vi "Poll.Main.vi"(8 "error in (no error)":errorcluster, 10 "Paramaters":variant, 11 "Process":refnum<class "Process.lvclass">) -> ()   [LabVIEW 2015, in "OPC UA Client Engine.lvlib"]
uses:
  OPC UA Client Engine.lvlib
  <vilib>/NI/NIVS Inline Async API/_VS Inline Async API/Process/Process.lvclass
  Types/Poll.Parameters.ctl
  Shared/Compiled.Settings.ctl
  Shared/OPCConnection.Properties.ctl
  Shared/Poll.ListProperties.ctl
  Shared/Tag.WriteProperties.Info.ctl
  Shared/Tags.ReadWriteRefs.ctl
  <vilib>/NI Veristand/Custom Device API/Data Reference.ctl
  <vilib>/NI Veristand/Custom Device API/Custom Device Target Type.ctl
  <vilib>/NI/NIVS Inline Async API/_Data Access Engine/Access Type Classes/Write/Write.lvclass/Write.ctl
  <vilib>/NI/NIVS Inline Async API/_VS Inline Async API/Process/Process.lvclass/Process.ctl
  Shared/DataRefs.Location.ctl
  <vilib>/NI/NIVS Inline Async API/_Data Access Engine/Data Access Engine/Methods/Write.Data.vi
  <vilib>/NI/NIVS Inline Async API/_VS Inline Async API/Error Handling Process/SubVIs/Error.ConvertArray.vi
  <vilib>/NI/NIVS Inline Async API/_Data Access Engine/Access Type Classes/Write/Write.ProcessData.vi
  <vilib>/OPCUA/client/Write DateTime Array.vi
  <vilib>/OPCUA/client/Write Double Array.vi
  <vilib>/OPCUA/client/Write Float Array.vi
  <vilib>/OPCUA/client/Write UInt64 Array.vi
  <vilib>/OPCUA/client/Write Int64 Array.vi
  <vilib>/OPCUA/client/Write UInt32 Array.vi
  <vilib>/OPCUA/client/Write Int32 Array.vi
  <vilib>/OPCUA/client/Write UInt16 Array.vi
  <vilib>/OPCUA/client/Write Int16 Array.vi
  <vilib>/OPCUA/client/Write Byte Array.vi
  <vilib>/OPCUA/client/Write SByte Array.vi
  <vilib>/OPCUA/client/Write Bool Array.vi
  <vilib>/OPCUA/client/Write DateTime.vi
  <vilib>/OPCUA/client/Write Double.vi
  <vilib>/OPCUA/client/Write Float.vi
  <vilib>/OPCUA/client/Write UInt64.vi
  <vilib>/OPCUA/client/Write Int64.vi
  <vilib>/OPCUA/client/Write UInt32.vi
  <vilib>/OPCUA/client/Write Int32.vi
  <vilib>/OPCUA/client/Write UInt16.vi
  <vilib>/OPCUA/client/Write Int16.vi
  <vilib>/OPCUA/client/Write Byte.vi
  <vilib>/OPCUA/client/Write SByte.vi
  <vilib>/OPCUA/client/Write Bool.vi
  <vilib>/OPCUA/NI OPC UA Client.lvlib
  Shared/OPC UA Client Shared.lvlib
  <vilib>/NI Veristand/Custom Device Tools/Custom Device Utility Library/Custom Device Utility Library.lvlib
  <vilib>/NI VeriStand/Custom Device API/Custom Device API.lvlib
  <vilib>/NI/NIVS Inline Async API/_Data Access Engine/Data Access Engine/Data Access Engine.lvclass
panel:
  out "Read Code":i32
  out "Write Code":i32
  out "Read Table":variant
  out "Write Table":variant
  out "error out":errorcluster
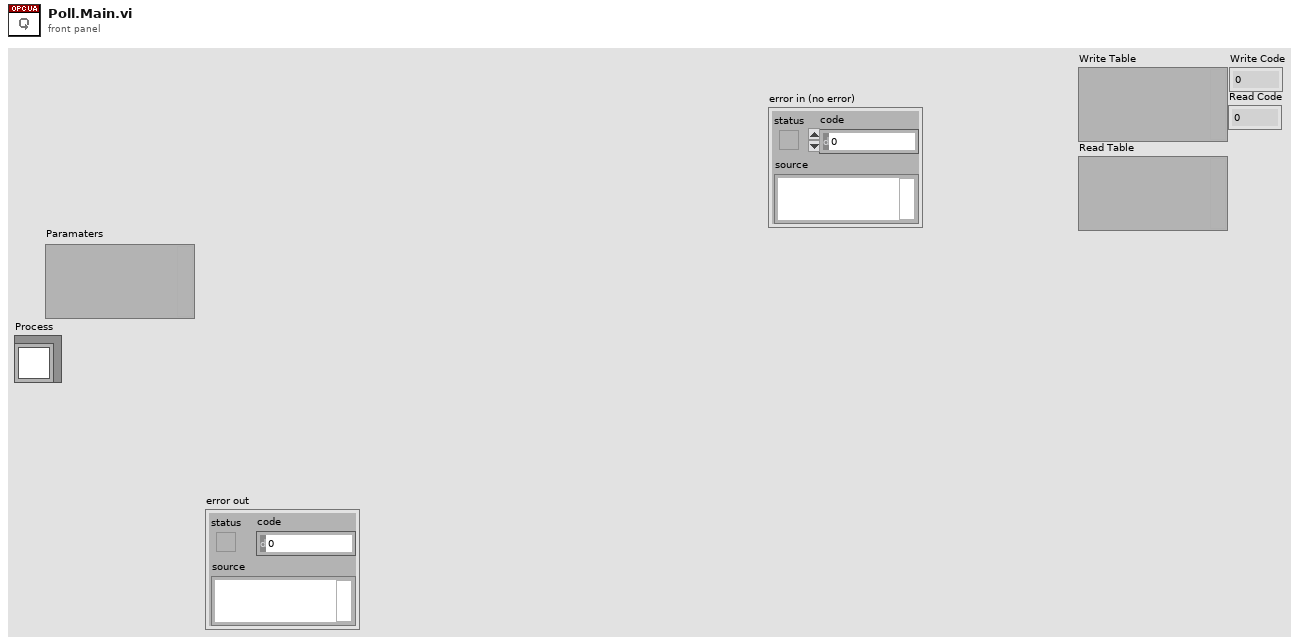
[diagram p1: front panel]
types:
  T1 = typedef "OPC UA Client Engine.lvlib/Poll.Parameters.ctl" = cluster{"Settings":T2, "WriteData":refnum<k33>, "ReadData":refnum<k33>, "WriteUpdate":refnum<k33>, "ReadUpdate":refnum<k33>, "Target Type":T8}
  T2 = typedef "OPC UA Client Shared.lvlib/Compiled.Settings.ctl" = cluster{"Connection.Properties":T3, "PollEngine.Settings":T4[], "LUT":variant, "Write Locations":T5[], "TotalTags":u32, "Data Refs":T6}
  T3 = typedef "OPC UA Client Shared.lvlib/OPCConnection.Properties.ctl" = cluster{"Server IP Address":string, "Server Port":u16, "Message Mode":enum16{"None", "Sign", "Sign and Encrypt"}, "Security":enum16{"Basic256", "Basic128Rsa15"}, "User Name":string, "Password":string, "Client Certificate":path, "Server Certificate":path, "Server Certificate (RT)":path, "Client Certificate (RT)":path}
  T4 = typedef "OPC UA Client Shared.lvlib/Poll.ListProperties.ctl" = cluster{"Poll Rate":dbl, "Tags":string[]}
  T5 = typedef "OPC UA Client Shared.lvlib/Tag.WriteProperties.Info.ctl" = cluster{"Path":string, "Offset":i32, "Length":i32, "DataType":u32}
  T6 = typedef "OPC UA Client Shared.lvlib/Tags.ReadWriteRefs.ctl" = cluster{"Read Refs":T7[], "Read Values":dbl[], "Read?":bool[], "Access":enum8{"Null", "Read", "Write", "Read&Write"}[], "Write Refs":T7[], "Write Values":dbl[], "Write?":bool[], "Write Only Location":u32, "Write? Reset":bool[]}
  T7 = typedef "Custom Device API.lvlib/Data Reference.ctl" = i32
  T8 = typedef "Custom Device API.lvlib/Custom Device Target Type.ctl" = enum16{"PharLap", "VxWorks", "Windows", "Linux_32_ARM", "Linux_x64"}
  T9 = typedef "OPC UA Client Shared.lvlib/DataRefs.Location.ctl" = cluster{"Offset":i32, "Length":i32}
  T10 = typedef "OPC UA Client Engine.lvlib/Poll.StateVariables.ctl" = cluster{"SubscriptionIDs":u32[], "OPCEvent":refnum<event-registration>, "Stop Ref":refnum<data-value>, "OPC UA client Ref":refnum<k21>, "Data Change":refnum<user-event>, "Process":refnum<class "Process.lvclass">, "Status Ref":T11}
  T11 = typedef "Data Access Engine.lvlib/Data Access Engine.lvclass/Write.DVR.ctl" = refnum<data-value>
  T12 = cluster{"Item URL":string, "Item Value":variant, "Timestamp":timestamp, "DataType":u32, "status code":u32}[]
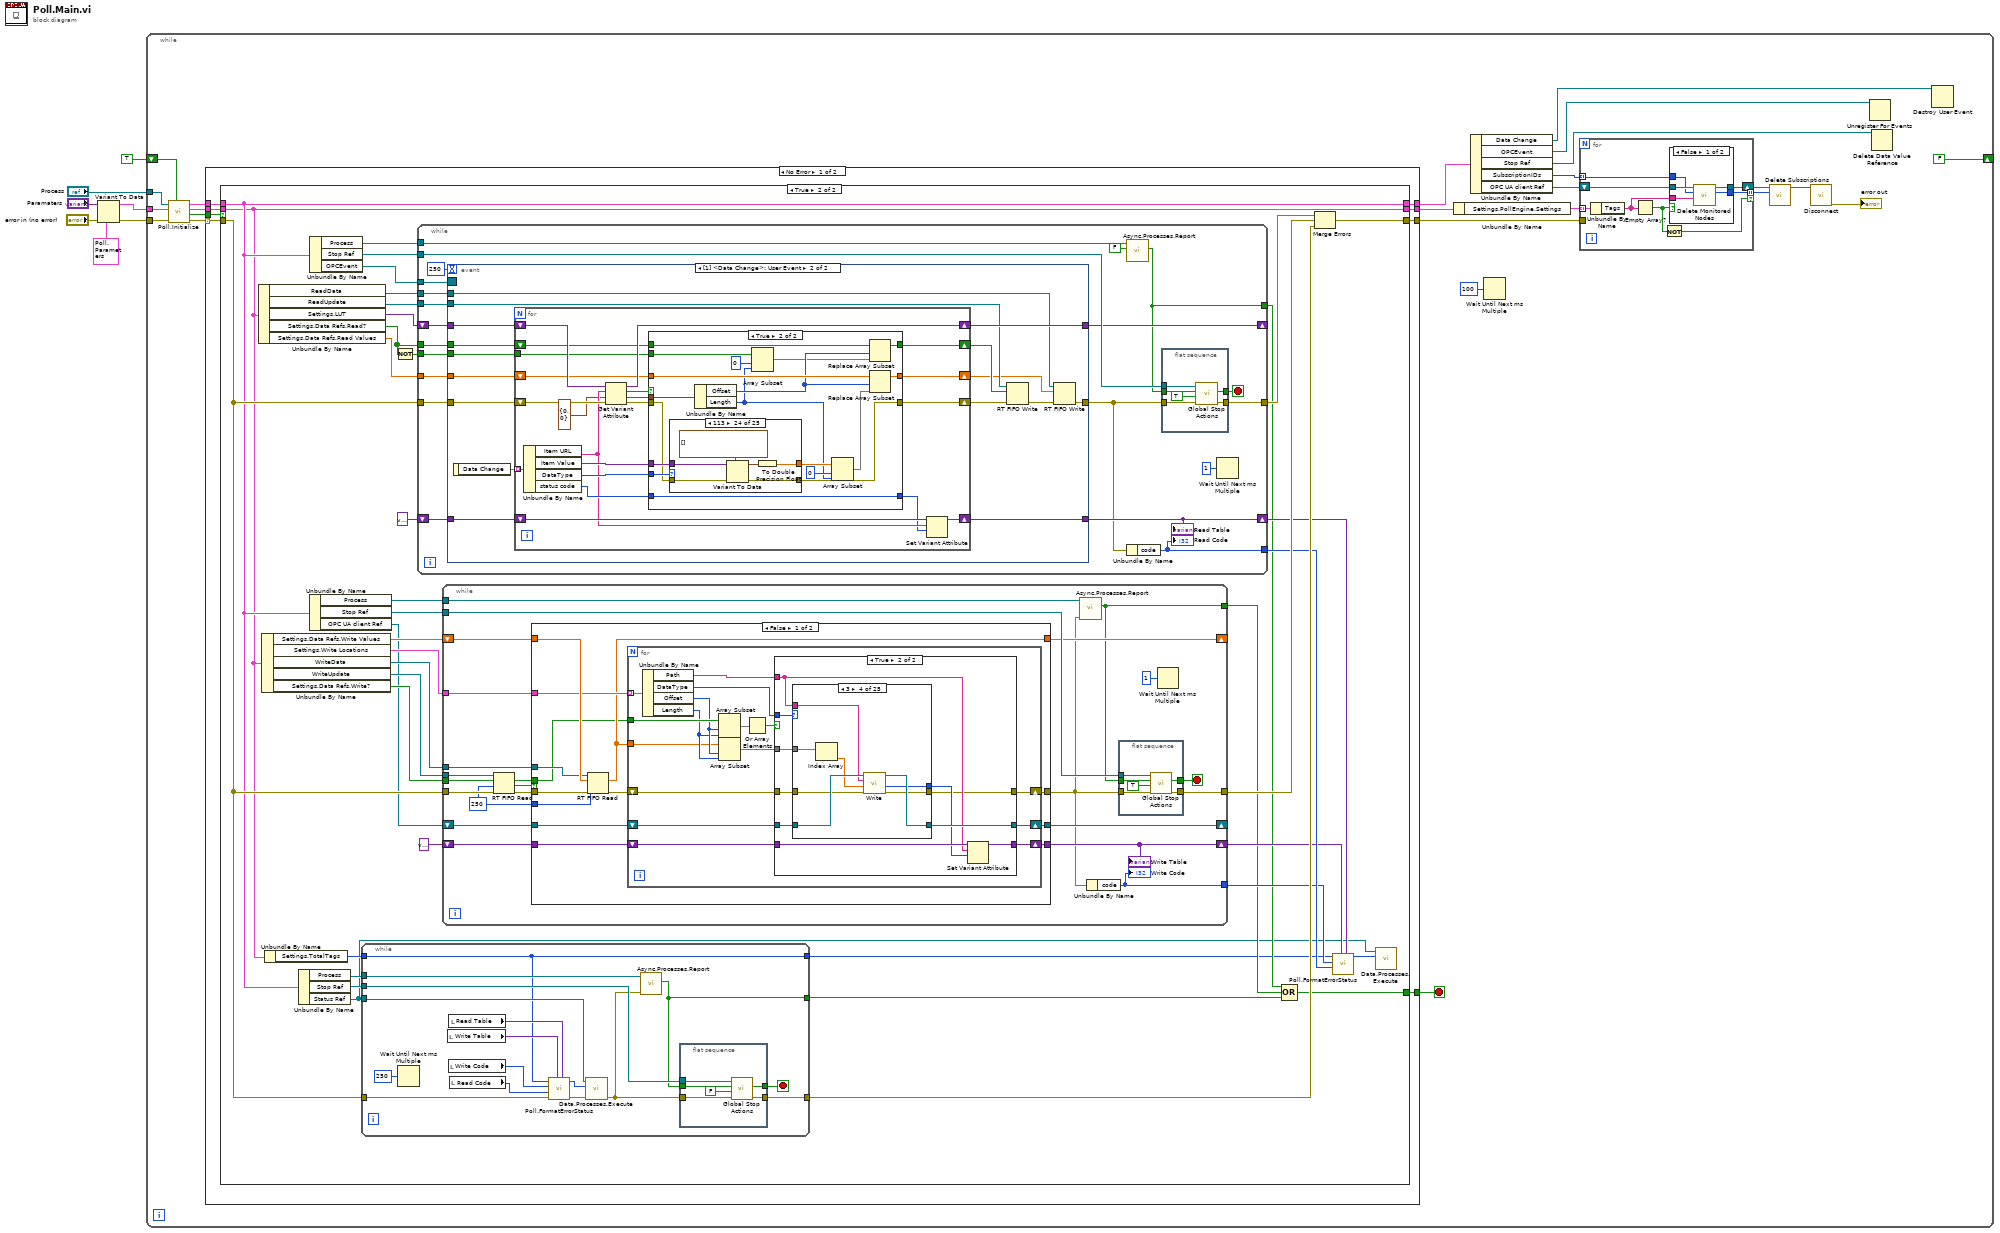
[diagram p0: block diagram]
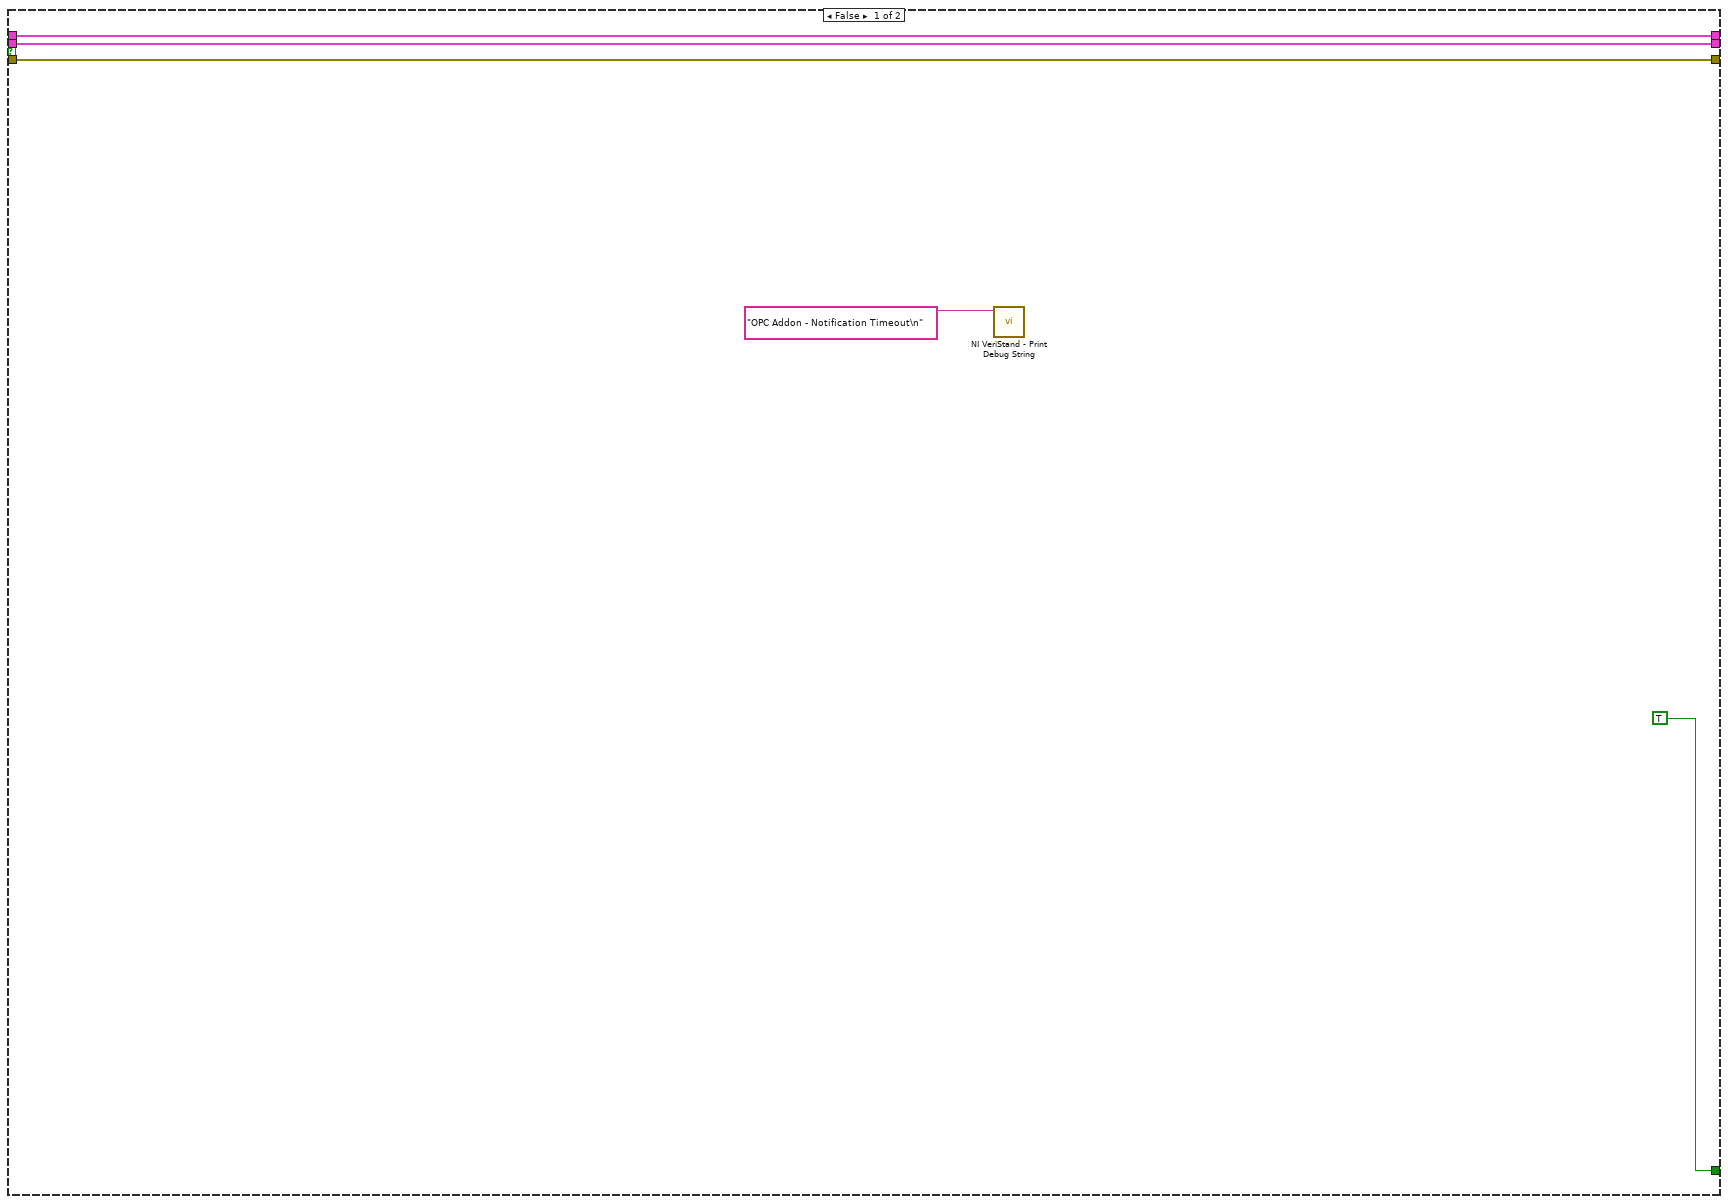
[diagram p2: hidden frame]
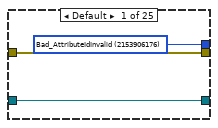
[diagram p4: hidden frame]
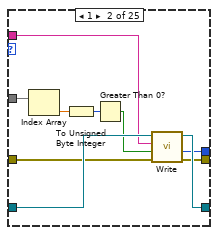
[diagram p5: hidden frame]
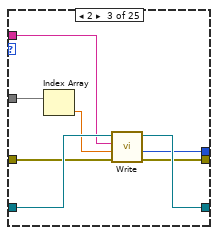
[diagram p6: hidden frame]
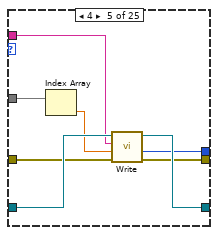
[diagram p7: hidden frame]
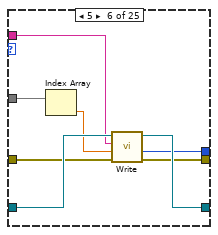
[diagram p8: hidden frame]
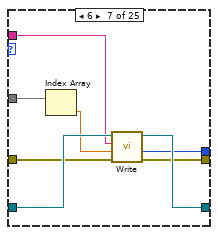
[diagram p9: hidden frame]
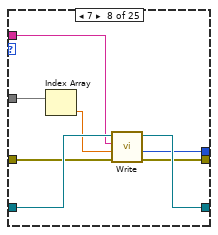
[diagram p10: hidden frame]
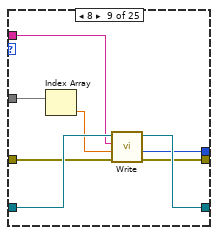
[diagram p11: hidden frame]
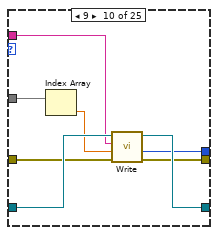
[diagram p12: hidden frame]
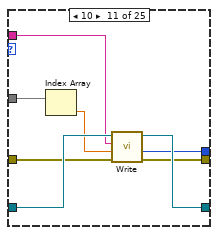
[diagram p13: hidden frame]
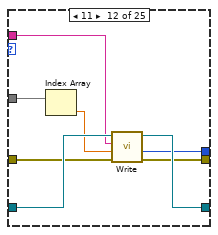
[diagram p14: hidden frame]
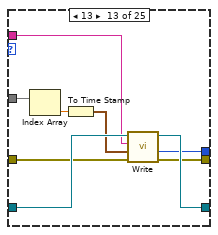
[diagram p15: hidden frame]
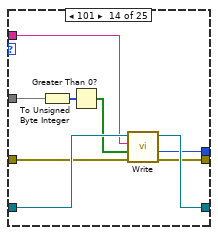
[diagram p16: hidden frame]
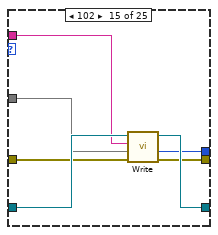
[diagram p17: hidden frame]
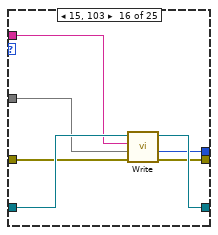
[diagram p18: hidden frame]
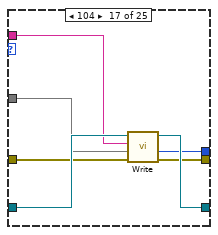
[diagram p19: hidden frame]
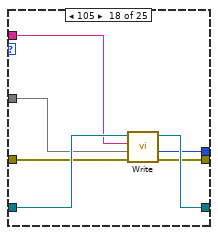
[diagram p20: hidden frame]
diagram:
  n1 = Variant To Data(error in="error in (no error)", type=T1 {"Settings"={"Connection.Properties"={"Server IP Address"="", "Server Port"=0, "Message Mode"=enum."None", "Security"=enum."Basic256", "User Name"="", "Password"="", "Client Certificate"=path "", "Server Certificate"=path "", "Server Certificate (RT)"=path "", "Client Certificate (RT)"=path ""}, "PollEngine.Settings"=[], "LUT"=variant, "Write Locations"=[], "TotalTags"=0, "Data Refs"={"Read Refs"=[], "Read Values"=[], "Read?"=[], "Access"=[], "Write Refs"=[], "Write Values"=[], "Write?"=[], "Write Only Location"=0, "Write? Reset"=[]}}, "WriteData"=refnum, "ReadData"=refnum, "WriteUpdate"=refnum, "ReadUpdate"=refnum, "Target Type"=enum."PharLap"} ("Parameters"), Variant="Paramaters") -> (data=w3:T1, error out=w4:errorcluster)
  n2 = while {
    tunnel: w4 -> [w13]
    tunnel: w3 -> [w12]
    shift-right: [FALSE] -> _
    shift-left: TRUE -> [w11]
    tunnel: "Process" -> [w8]
    stop <- w9 stop-if-true
    n3 = call "Poll.Initialize.vi"("FirstCall?"=w11, "error in (no error)"=w13, "Parameters in"=w12, "Process"=w8) -> ("error out"=w15:errorcluster, "notification"=w27:bool, "Parameters out"=w28:T1, "Settings"=w26:T10)  [unwired: 4 in]
    n4 = case shown="No Error" w15 {
      selector: w15 -> [w33 w620]
      tunnel: [w39 w620] -> w30
      tunnel: w28 -> [w38 w624]
      tunnel: w27 -> [w37 _]
      tunnel: w26 -> [w36 w622]
      tunnel: [w35 w624] -> w25
      tunnel: [w34 w622] -> w23
      tunnel: [w32 w619] -> w9
      frame No Error {
        n5 = case shown="True" w37 {
          tunnel: w36 -> [w43 w82]
          tunnel: w33 -> [w44 w84]
          tunnel: [w44 w83] -> w39
          tunnel: w38 -> [w42 w81]
          tunnel: [w43 w82] -> w34
          tunnel: [w42 w81] -> w35
          tunnel: [TRUE w48] -> w32
          frame False {
            n6 = call <vilib>:"NI VeriStand - Print Debug String.vi"("Message"="OPC Addon - Notification Timeout\n") -> ()  [unwired: 10 in, 1 out]
          }
          frame True {
            n7 = Unbundle By Name(w81) -> ("ReadData"=w74:refnum<k33>, "ReadUpdate"=w61:refnum<k33>, "Settings.LUT"=w73:variant, "Settings.Data Refs.Read?"=w60:bool[], "Settings.Data Refs.Read Values"=w58:dbl[])
            n8 = Unbundle By Name(w81) -> ("Settings.Data Refs.Write Values"=w77:dbl[], "Settings.Write Locations"=w76:T5[], "WriteData"=w75:refnum<k33>, "WriteUpdate"=w63:refnum<k33>, "Settings.Data Refs.Write?"=w62:bool[])
            n9 = Unbundle By Name(w81) -> ("Settings.TotalTags"=w47:u32)
            n10 = Unbundle By Name(w82) -> ("Process"=w66:refnum<class "Process.lvclass">, "Stop Ref"=w69:refnum<data-value>, "Status Ref"=w46:T11)
            n11 = Unbundle By Name(w82) -> ("Process"=w65:refnum<class "Process.lvclass">, "Stop Ref"=w70:refnum<data-value>, "OPC UA client Ref"=w57:refnum<k21>)
            n12 = Unbundle By Name(w82) -> ("Process"=w64:refnum<class "Process.lvclass">, "Stop Ref"=w71:refnum<data-value>, "OPCEvent"=w72:refnum<event-registration>)
            n13 = while {
              tunnel: w84 -> [w100]
              tunnel: w69 -> [w99]
              tunnel: [w96] -> w68
              tunnel: w66 -> [w95]
              tunnel: [w87] -> w51
              tunnel: w46 -> [w86]
              tunnel: w47 -> [w85]
              tunnel: [w85] -> w45
              stop <- w89 stop-if-true
              n14 = Wait Until Next ms Multiple(millisecond multiple=u32 250) -> ()  [unwired: 1 out]
              n15 = local read "Write Table"() -> (w91:variant)
              n16 = local read "Write Code"() -> (w94:i32)
              n17 = local read "Read Table"() -> (w90:variant)
              n18 = local read "Read Code"() -> (w93:i32)
              n19 = call "Poll.FormatErrorStatus.vi"("Read Table"=w90, "Write Table"=w91, "error in (no error)"=w100, "Read Code"=w93, "Write Code"=w94, "TotalTags"=w85) -> ("error out"=w98:errorcluster, "ErrorStatus"=w97:u32[])  [unwired: 4 in]
              n20 = call-poly <vilib>:"Data.Processes.Execute.vi"("error in (no error)"=w98, "Values"=w97, "Ref"=w86) -> ("error out"=w88:errorcluster)  [unwired: 8 in]
              n21 = call <vilib>:"Async.Processes.Report.vi"("Error"=w88, "Process in"=w95) -> ("Stop"=w87:bool)  [unwired: 8 in, 1 out]
              n22 = flat-sequence {
                tunnel: w99 -> [w105]
                tunnel: [w104] -> w89
                tunnel: w88 -> [w103]
                tunnel: [w102] -> w96
                tunnel: w87 -> [w101]
                frame #0 {
                  n23 = call "Global Stop Actions.vi"("error in (no error)"=w103, "Stop on Error?"=FALSE, "Stop?"=w101, "Stop Ref"=w105) -> ("error out"=w102:errorcluster, "Latched Stop"=w104:bool)  [unwired: 5 in, 1 out]
                }
              }
            }
            n24 = Not(x=w60) -> (.not. x?=w59:bool[])
            n25 = while {
              tunnel: w72 -> [w391]
              shift-right: [w385] -> _
              shift-left: w73 -> [w388]
              tunnel: w74 -> [w380]
              tunnel: w84 -> [w389]
              tunnel: [w382] -> w67
              shift-right: [w384] -> w55
              shift-left: variant ("variant") -> [w387]
              tunnel: w71 -> [w386]
              tunnel: w64 -> [w381]
              tunnel: w61 -> [w379]
              tunnel: w60 -> [w378]
              tunnel: w59 -> [w377]
              tunnel: [w375] -> w54
              tunnel: w58 -> [w376]
              tunnel: [w372] -> w49
              stop <- w374 stop-if-true
              n26 = event shown="[1] <Data Change>: User Event" {
                selector: w391 -> [_ _]
                dyn-events: _ -> [_ _]
                timeout: 250 -> [_ _]
                tunnel: w389 -> [w400 w413]
                tunnel: [w400 w409] -> w371
                tunnel: w388 -> [w399 w415]
                tunnel: [w399 w414] -> w385
                tunnel: w387 -> [w398 w412]
                tunnel: [w398 w411] -> w384
                tunnel: w376 -> [_ w410]
                tunnel: w380 -> [_ w408]
                tunnel: w379 -> [_ w405]
                tunnel: w378 -> [_ w403]
                tunnel: w377 -> [_ w402]
                event Timeout {
                  n27 = event-data() -> ()  [unwired: 1 in, 2 out]
                }
                event User Event {
                  n28 = event-data() -> ("Data Change"=w416:T12)  [unwired: 1 in]
                  n29 = for {
                    tunnel: w416 -> [w437] mode=indexing
                    shift-right: [w433] -> w414
                    shift-left: w415 -> [w435]
                    shift-right: [w417] -> w407
                    shift-left: w413 -> [w432]
                    shift-right: [w424] -> w411
                    shift-left: w412 -> [w427]
                    shift-right: [w421] -> w401
                    shift-left: w410 -> [w422]
                    shift-right: [w419] -> w404
                    shift-left: w403 -> [w420]
                    tunnel: w402 -> [w418]
                    n30 = Unbundle By Name(w437) -> ("Item URL"=w426:string, "Item Value"=w436:variant, "DataType"=w431:u32, "status code"=w429:u32)
                    n31 = Get Variant Attribute(Variant=w435, name=w426, default value (empty Variant)=T9 {"Offset"=0, "Length"=0} ("cluster"), error in=w432) -> (duplicate Variant=w433:variant, found=w428:bool, value=w434:T9, error out=w430:errorcluster)
                    n32 = case shown="True" w428 {
                      tunnel: w436 -> [_ w459]
                      tunnel: w434 -> [_ w454]
                      tunnel: [w441 w453] -> w417
                      tunnel: w431 -> [_ w458]
                      tunnel: w430 -> [w441 w457]
                      tunnel: w429 -> [_ w456]
                      tunnel: [w440 w456] -> w425
                      tunnel: w422 -> [w439 w455]
                      tunnel: [w439 w450] -> w421
                      tunnel: w420 -> [w438 w446]
                      tunnel: [w438 w447] -> w419
                      tunnel: w418 -> [_ w443]
                      frame False {
                        w440 = u32 2153906176 items=["Good"=0, "Bad_AttributeIdInvalid"=2153906176, "Bad_BrowseDirectionInvalid"=2152529920, "Bad_BrowseNameInvalid"=2153775104, "Bad_ContentFilterInvalid"=2152202240, "Bad_ContinuationPointInvalid"=2152333312, "Bad_DataEncodingInvalid"=2151153664, "Bad_DataEncodingUnsupported"=2151219200, "Bad_EventFilterInvalid"=2152136704, "Bad_FilterNotAllowed"=2152005632, "Bad_FilterOperandInvalid"=2160132096, "Bad_HistoryOperationInvalid"=2154889216, "Bad_HistoryOperationUnsupported"=2154954752, "Bad_IndexRangeInvalid"=2151022592, "Bad_IndexRangeNoData"=2151088128, "Bad_MonitoredItemFilterInvalid"=2151874560, "Bad_MonitoredItemFilterUnsupported"=2151940096, "Bad_MonitoredItemIdInvalid"=2151809024, "Bad_MonitoringModeInvalid"=2151743488, "Bad_NoCommunication"=2150694912, "Bad_NoContinuationPoints"=2152398848, "Bad_NodeClassInvalid"=2153709568, "Bad_NodeIdInvalid"=2150825984, "Bad_NodeIdUnknown"=2150891520, "Bad_NoDeleteRights"=2154364928, "Bad_NodeNotInView"=2152595456, "Bad_NotFound"=2151546880, "Bad_NotImplemented"=2151677952, "Bad_NotReadable"=2151284736, "Bad_NotSupported"=2151481344, "Bad_NotWritable"=2151350272, "Bad_ObjectDeleted"=2151612416, "Bad_OutOfRange"=2151415808, "Bad_ReferenceTypeIdInvalid"=2152464384, "Bad_SourceNodeIdInvalid"=2154037248, "Bad_StructureMissing"=2152071168, "Bad_TargetNodeIdInvalid"=2154102784, "Bad_TypeDefinitionInvalid"=2153971712, "Bad_TypeMismatch"=2155085824, "Bad_WaitingForInitialData"=2150760448] ("status")
                      }
                      frame True {
                        n33 = case shown="113" w458 {
                          tunnel: w459 -> [w467 w474 w481 w488 w495 w502 w509 w516 w523 w530 w537 w544 w551 w557 w563 w569 w575 w581 w587 w593 w599 w605 w611 w617 _]
                          tunnel: w457 -> [w466 w473 w480 w487 w494 w501 w508 w515 w522 w529 w536 w543 w550 w556 w562 w568 w574 w580 w586 w592 w598 w604 w610 w616 w618]
                          tunnel: [w465 w472 w479 w486 w493 w500 w507 w514 w521 w528 w535 w542 w549 w555 w561 w567 w573 w579 w585 w591 w597 w603 w609 w615 w618] -> w453
                          tunnel: [w460 w469 w476 w483 w490 w497 w504 w511 w518 w525 w532 w539 w545 w553 w559 w565 w571 w577 w583 w589 w595 w601 w607 w613 _] -> w452
                          frame 1 {
                            n34 = Variant To Data(error in=w466, type=FALSE, Variant=w467) -> (data=w463:bool, error out=w465:errorcluster)
                            n35 = Boolean To (0,1)(Boolean=w463) -> (0, 1=w462:i16)
                            n36 = To Double Precision Float(number=w462) -> (double precision float=w461:dbl)
                            n37 = Build Array(w461) -> (w460:dbl[])
                          }
                          frame 2 {
                            n38 = Variant To Data(error in=w473, type=i8 0, Variant=w474) -> (data=w468:i8, error out=w472:errorcluster)
                            n39 = To Double Precision Float(number=w468) -> (double precision float=w470:dbl)
                            n40 = Build Array(w470) -> (w469:dbl[])
                          }
                          frame 3 {
                            n41 = Variant To Data(error in=w480, type=u8 0, Variant=w481) -> (data=w475:u8, error out=w479:errorcluster)
                            n42 = To Double Precision Float(number=w475) -> (double precision float=w477:dbl)
                            n43 = Build Array(w477) -> (w476:dbl[])
                          }
                          frame 4 {
                            n44 = Variant To Data(error in=w487, type=i16 0, Variant=w488) -> (data=w482:i16, error out=w486:errorcluster)
                            n45 = To Double Precision Float(number=w482) -> (double precision float=w484:dbl)
                            n46 = Build Array(w484) -> (w483:dbl[])
                          }
                          frame 5 {
                            n47 = Variant To Data(error in=w494, type=u16 0, Variant=w495) -> (data=w489:u16, error out=w493:errorcluster)
                            n48 = To Double Precision Float(number=w489) -> (double precision float=w491:dbl)
                            n49 = Build Array(w491) -> (w490:dbl[])
                          }
                          frame 6 {
                            n50 = Variant To Data(error in=w501, type=0, Variant=w502) -> (data=w496:i32, error out=w500:errorcluster)
                            n51 = To Double Precision Float(number=w496) -> (double precision float=w498:dbl)
                            n52 = Build Array(w498) -> (w497:dbl[])
                          }
                          frame 7 {
                            n53 = Variant To Data(error in=w508, type=u32 0, Variant=w509) -> (data=w503:u32, error out=w507:errorcluster)
                            n54 = To Double Precision Float(number=w503) -> (double precision float=w505:dbl)
                            n55 = Build Array(w505) -> (w504:dbl[])
                          }
                          frame 8 {
                            n56 = Variant To Data(error in=w515, type=i64 0, Variant=w516) -> (data=w510:i64, error out=w514:errorcluster)
                            n57 = To Double Precision Float(number=w510) -> (double precision float=w512:dbl)
                            n58 = Build Array(w512) -> (w511:dbl[])
                          }
                          frame 9 {
                            n59 = Variant To Data(error in=w522, type=u64 0, Variant=w523) -> (data=w517:u64, error out=w521:errorcluster)
                            n60 = To Double Precision Float(number=w517) -> (double precision float=w519:dbl)
                            n61 = Build Array(w519) -> (w518:dbl[])
                          }
                          frame 10 {
                            n62 = Variant To Data(error in=w529, type=sgl 0.0, Variant=w530) -> (data=w524:sgl, error out=w528:errorcluster)
                            n63 = To Double Precision Float(number=w524) -> (double precision float=w526:dbl)
                            n64 = Build Array(w526) -> (w525:dbl[])
                          }
                          frame 11 {
                            n65 = Variant To Data(error in=w536, type=0.0, Variant=w537) -> (data=w531:dbl, error out=w535:errorcluster)
                            n66 = To Double Precision Float(number=w531) -> (double precision float=w533:dbl)
                            n67 = Build Array(w533) -> (w532:dbl[])
                          }
                          frame 13 {
                            n68 = Variant To Data(error in=w543, type=timestamp(0 s since 1904-01-01), Variant=w544) -> (data=w538:timestamp, error out=w542:errorcluster)
                            n69 = To Double Precision Float(number=w538) -> (double precision float=w540:dbl)
                            n70 = Build Array(w540) -> (w539:dbl[])
                          }
                          frame 101 {
                            n71 = Variant To Data(error in=w550, type=bool[] [], Variant=w551) -> (data=w548:bool[], error out=w549:errorcluster)
                            n72 = Boolean To (0,1)(Boolean=w548) -> (0, 1=w547:i16[])
                            n73 = To Double Precision Float(number=w547) -> (double precision float=w545:dbl[])
                          }
                          frame 102 {
                            n74 = Variant To Data(error in=w556, type=i8[] [], Variant=w557) -> (data=w552:i8[], error out=w555:errorcluster)
                            n75 = To Double Precision Float(number=w552) -> (double precision float=w553:dbl[])
                          }
                          frame 15, 103 {
                            n76 = Variant To Data(error in=w562, type=u8[] [], Variant=w563) -> (data=w558:u8[], error out=w561:errorcluster)
                            n77 = To Double Precision Float(number=w558) -> (double precision float=w559:dbl[])
                          }
                          frame 104 {
                            n78 = Variant To Data(error in=w568, type=i16[] [], Variant=w569) -> (data=w564:i16[], error out=w567:errorcluster)
                            n79 = To Double Precision Float(number=w564) -> (double precision float=w565:dbl[])
                          }
                          frame 105 {
                            n80 = Variant To Data(error in=w574, type=u16[] [], Variant=w575) -> (data=w570:u16[], error out=w573:errorcluster)
                            n81 = To Double Precision Float(number=w570) -> (double precision float=w571:dbl[])
                          }
                          frame 106 {
                            n82 = Variant To Data(error in=w580, type=i32[] [], Variant=w581) -> (data=w576:i32[], error out=w579:errorcluster)
                            n83 = To Double Precision Float(number=w576) -> (double precision float=w577:dbl[])
                          }
                          frame 107 {
                            n84 = Variant To Data(error in=w586, type=u32[] [], Variant=w587) -> (data=w582:u32[], error out=w585:errorcluster)
                            n85 = To Double Precision Float(number=w582) -> (double precision float=w583:dbl[])
                          }
                          frame 108 {
                            n86 = Variant To Data(error in=w592, type=i64[] [], Variant=w593) -> (data=w588:i64[], error out=w591:errorcluster)
                            n87 = To Double Precision Float(number=w588) -> (double precision float=w589:dbl[])
                          }
                          frame 109 {
                            n88 = Variant To Data(error in=w598, type=u64[] [], Variant=w599) -> (data=w594:u64[], error out=w597:errorcluster)
                            n89 = To Double Precision Float(number=w594) -> (double precision float=w595:dbl[])
                          }
                          frame 110 {
                            n90 = Variant To Data(error in=w604, type=sgl[] [], Variant=w605) -> (data=w600:sgl[], error out=w603:errorcluster)
                            n91 = To Double Precision Float(number=w600) -> (double precision float=w601:dbl[])
                          }
                          frame 111 {
                            n92 = Variant To Data(error in=w610, type=dbl[] [], Variant=w611) -> (data=w606:dbl[], error out=w609:errorcluster)
                            n93 = To Double Precision Float(number=w606) -> (double precision float=w607:dbl[])
                          }
                          frame 113 {
                            n94 = Variant To Data(error in=w616, type=timestamp[] [], Variant=w617) -> (data=w612:timestamp[], error out=w615:errorcluster)
                            n95 = To Double Precision Float(number=w612) -> (double precision float=w613:dbl[])
                          }
                          frame Default {
                          }
                        }
                        n96 = Unbundle By Name(w454) -> ("Offset"=w449:i32, "Length"=w445:i32)
                        n97 = Array Subset(array=w443, index=0, length=w445) -> (w442:bool[])
                        n98 = Array Subset(array=w452, index=0, length=w445) -> (w451:dbl[])
                        n99 = Replace Array Subset(array=w446, new element=w442, index=w449) -> (w447:bool[])
                        n100 = Replace Array Subset(array=w455, new element=w451, index=w449) -> (w450:dbl[])
                      }
                    }
                    n101 = Set Variant Attribute(Variant=w427, name=w426, value=w425) -> (Variant out=w424:variant)  [unwired: 1 in, 2 out]
                  }
                  n102 = RT FIFO Write(0:w405, 1:w404, 3:w407) -> (11:w406:errorcluster)  [unwired: 2 in, 3 out]
                  n103 = RT FIFO Write(0:w408, 1:w401, 3:w406) -> (11:w409:errorcluster)  [unwired: 2 in, 3 out]
                }
              }
              "Read Table" <- w384
              n104 = call <vilib>:"Async.Processes.Report.vi"("Stop Async on Error?"=FALSE ("Stop on Error?"), "Process in"=w381) -> ("Stop"=w372:bool)  [unwired: 8 in, 1 out]
              n105 = Unbundle By Name(w371) -> ("code"=w375:i32)
              "Read Code" <- w375
              n106 = flat-sequence {
                tunnel: w371 -> [w397]
                tunnel: w386 -> [w395]
                tunnel: [w394] -> w382
                tunnel: [w393] -> w374
                tunnel: w372 -> [w392]
                frame #0 {
                  n107 = call "Global Stop Actions.vi"("error in (no error)"=w397, "Stop on Error?"=TRUE, "Stop?"=w392, "Stop Ref"=w395) -> ("error out"=w394:errorcluster, "Latched Stop"=w393:bool)  [unwired: 5 in, 1 out]
                }
              }
              n108 = Wait Until Next ms Multiple(millisecond multiple=u32 1) -> ()  [unwired: 1 out]
            }
            n109 = while {
              tunnel: w76 -> [w128]
              shift-right: [w120] -> _
              shift-left: w77 -> [w129]
              tunnel: w75 -> [w126]
              tunnel: w84 -> [w119]
              tunnel: [w121] -> w78
              shift-right: [w125] -> _
              shift-left: w57 -> [w127]
              shift-right: [w124] -> w52
              shift-left: variant ("variant") -> [w123]
              tunnel: w70 -> [w122]
              tunnel: w65 -> [w109]
              tunnel: w63 -> [w117]
              tunnel: w62 -> [w116]
              tunnel: [w111] -> w53
              tunnel: [w108] -> w50
              stop <- w110 stop-if-true
              w115 = 250 ("timeout in ms (0)")
              n110 = RT FIFO Read(0:w117, 1:w116, 2:w115, 3:w119) -> (9:w114:bool[], 10:w113:bool, 11:w118:errorcluster)  [unwired: 2 out]
              n111 = case shown="False" w113 {
                tunnel: w129 -> [w147 w370]
                tunnel: w128 -> [w146 _]
                tunnel: w127 -> [w145 w367]
                tunnel: w126 -> [w144 _]
                tunnel: [w143 w367] -> w125
                tunnel: [w142 w368] -> w124
                tunnel: w123 -> [w141 w368]
                tunnel: [w140 w369] -> w107
                tunnel: [w139 w370] -> w120
                tunnel: w118 -> [w138 w369]
                tunnel: w115 -> [w137 _]
                tunnel: w114 -> [w136 _]
                frame False {
                  n112 = RT FIFO Read(0:w144, 1:w147, 2:w137, 3:w138) -> (9:w139:dbl[], 11:w148:errorcluster)  [unwired: 3 out]
                  n113 = for {
                    tunnel: w136 -> [w160]
                    tunnel: w146 -> [w158] mode=indexing
                    shift-right: [w162] -> w140
                    shift-left: w148 -> [w161]
                    shift-right: [w163] -> w143
                    shift-left: w145 -> [w164]
                    tunnel: w139 -> [w154]
                    shift-right: [w152] -> w142
                    shift-left: w141 -> [w153]
                    n114 = Unbundle By Name(w158) -> ("Path"=w151:string, "DataType"=w155:u32, "Offset"=w157:i32, "Length"=w156:i32)
                    n115 = Array Subset(array=w160, index=w157, length=w156) -> (w149:bool[])
                    n116 = Array Subset(array=w154, index=w157, length=w156) -> (w159:dbl[])
                    n117 = Or Array Elements(Boolean array=w149) -> (logical OR=w150:bool)
                    n118 = case shown="True" w150 {
                      tunnel: w164 -> [w166 w177]
                      tunnel: [w166 w176] -> w163
                      tunnel: [w167 w168] -> w162
                      tunnel: w161 -> [w167 w175]
                      tunnel: w151 -> [_ w169]
                      tunnel: w159 -> [_ w174]
                      tunnel: w155 -> [_ w173]
                      tunnel: w153 -> [w165 w172]
                      tunnel: [w165 w170] -> w152
                      frame False {
                      }
                      frame True {
                        n119 = case shown="3" w173 {
                          tunnel: w177 -> [w180 w190 w198 w206 w214 w222 w230 w238 w246 w254 w262 w270 w279 w288 w295 w302 w309 w316 w323 w330 w337 w344 w351 w358 w366]
                          tunnel: [w180 w189 w197 w205 w213 w221 w229 w237 w245 w253 w261 w269 w278 w287 w294 w301 w308 w315 w322 w329 w336 w343 w350 w357 w365] -> w176
                          tunnel: [w179 w188 w196 w204 w212 w220 w228 w236 w244 w252 w260 w268 w277 w286 w293 w300 w307 w314 w321 w328 w335 w342 w349 w356 w364] -> w168
                          tunnel: w175 -> [w179 w187 w195 w203 w211 w219 w227 w235 w243 w251 w259 w267 w276 w285 w292 w299 w306 w313 w320 w327 w334 w341 w348 w355 w363]
                          tunnel: w174 -> [_ w185 w193 w201 w209 w217 w225 w233 w241 w249 w257 w265 w274 w283 w291 w298 w305 w312 w319 w326 w333 w340 w347 w354 w362]
                          tunnel: w169 -> [_ w182 w192 w200 w208 w216 w224 w232 w240 w248 w256 w264 w272 w281 w290 w297 w304 w311 w318 w325 w332 w339 w346 w353 w361]
                          tunnel: [w178 w181 w191 w199 w207 w215 w223 w231 w239 w247 w255 w263 w271 w280 w289 w296 w303 w310 w317 w324 w331 w338 w345 w352 w359] -> w171
                          frame Default {
                            w178 = u32 2153906176 items=["Good"=0, "Bad_AttributeIdInvalid"=2153906176, "Bad_BrowseDirectionInvalid"=2152529920, "Bad_BrowseNameInvalid"=2153775104, "Bad_ContentFilterInvalid"=2152202240, "Bad_ContinuationPointInvalid"=2152333312, "Bad_DataEncodingInvalid"=2151153664, "Bad_DataEncodingUnsupported"=2151219200, "Bad_EventFilterInvalid"=2152136704, "Bad_FilterNotAllowed"=2152005632, "Bad_FilterOperandInvalid"=2160132096, "Bad_HistoryOperationInvalid"=2154889216, "Bad_HistoryOperationUnsupported"=2154954752, "Bad_IndexRangeInvalid"=2151022592, "Bad_IndexRangeNoData"=2151088128, "Bad_MonitoredItemFilterInvalid"=2151874560, "Bad_MonitoredItemFilterUnsupported"=2151940096, "Bad_MonitoredItemIdInvalid"=2151809024, "Bad_MonitoringModeInvalid"=2151743488, "Bad_NoCommunication"=2150694912, "Bad_NoContinuationPoints"=2152398848, "Bad_NodeClassInvalid"=2153709568, "Bad_NodeIdInvalid"=2150825984, "Bad_NodeIdUnknown"=2150891520, "Bad_NoDeleteRights"=2154364928, "Bad_NodeNotInView"=2152595456, "Bad_NotFound"=2151546880, "Bad_NotImplemented"=2151677952, "Bad_NotReadable"=2151284736, "Bad_NotSupported"=2151481344, "Bad_NotWritable"=2151350272, "Bad_ObjectDeleted"=2151612416, "Bad_OutOfRange"=2151415808, "Bad_ReferenceTypeIdInvalid"=2152464384, "Bad_SourceNodeIdInvalid"=2154037248, "Bad_StructureMissing"=2152071168, "Bad_TargetNodeIdInvalid"=2154102784, "Bad_TypeDefinitionInvalid"=2153971712, "Bad_TypeMismatch"=2155085824, "Bad_WaitingForInitialData"=2150760448] ("status")
                          }
                          frame 1 {
                            n120 = Index Array(array=w185) -> (element=w186:dbl)  [unwired: 1 in]
                            n121 = To Unsigned Byte Integer(number=w186) -> (unsigned 8bit integer=w183:u8)
                            n122 = Greater Than 0?(x=w183) -> (x > 0?=w184:bool)
                            n123 = call-poly <vilib>:"Write.vi"("error in (no error)"=w187, "value"=w184, "node path"=w182, "OPC UA client refnum in"=w190) -> ("error out"=w188:errorcluster, "status"=w181:u32, "OPC UA client refnum out"=w189:refnum<k21>)  [unwired: 5 in]
                          }
                          frame 2 {
                            n124 = Index Array(array=w193) -> (element=w194:dbl)  [unwired: 1 in]
                            n125 = call-poly <vilib>:"Write.vi"("error in (no error)"=w195, "value"=w194, "node path"=w192, "OPC UA client refnum in"=w198) -> ("error out"=w196:errorcluster, "status"=w191:u32, "OPC UA client refnum out"=w197:refnum<k21>)  [unwired: 5 in]
                          }
                          frame 3 {
                            n126 = Index Array(array=w201) -> (element=w202:dbl)  [unwired: 1 in]
                            n127 = call-poly <vilib>:"Write.vi"("error in (no error)"=w203, "value"=w202, "node path"=w200, "OPC UA client refnum in"=w206) -> ("error out"=w204:errorcluster, "status"=w199:u32, "OPC UA client refnum out"=w205:refnum<k21>)  [unwired: 5 in]
                          }
                          frame 4 {
                            n128 = Index Array(array=w209) -> (element=w210:dbl)  [unwired: 1 in]
                            n129 = call-poly <vilib>:"Write.vi"("error in (no error)"=w211, "value"=w210, "node path"=w208, "OPC UA client refnum in"=w214) -> ("error out"=w212:errorcluster, "status"=w207:u32, "OPC UA client refnum out"=w213:refnum<k21>)  [unwired: 5 in]
                          }
                          frame 5 {
                            n130 = Index Array(array=w217) -> (element=w218:dbl)  [unwired: 1 in]
                            n131 = call-poly <vilib>:"Write.vi"("error in (no error)"=w219, "value"=w218, "node path"=w216, "OPC UA client refnum in"=w222) -> ("error out"=w220:errorcluster, "status"=w215:u32, "OPC UA client refnum out"=w221:refnum<k21>)  [unwired: 5 in]
                          }
                          frame 6 {
                            n132 = Index Array(array=w225) -> (element=w226:dbl)  [unwired: 1 in]
                            n133 = call-poly <vilib>:"Write.vi"("error in (no error)"=w227, "value"=w226, "node path"=w224, "OPC UA client refnum in"=w230) -> ("error out"=w228:errorcluster, "status"=w223:u32, "OPC UA client refnum out"=w229:refnum<k21>)  [unwired: 5 in]
                          }
                          frame 7 {
                            n134 = Index Array(array=w233) -> (element=w234:dbl)  [unwired: 1 in]
                            n135 = call-poly <vilib>:"Write.vi"("error in (no error)"=w235, "value"=w234, "node path"=w232, "OPC UA client refnum in"=w238) -> ("error out"=w236:errorcluster, "status"=w231:u32, "OPC UA client refnum out"=w237:refnum<k21>)  [unwired: 5 in]
                          }
                          frame 8 {
                            n136 = Index Array(array=w241) -> (element=w242:dbl)  [unwired: 1 in]
                            n137 = call-poly <vilib>:"Write.vi"("error in (no error)"=w243, "value"=w242, "node path"=w240, "OPC UA client refnum in"=w246) -> ("error out"=w244:errorcluster, "status"=w239:u32, "OPC UA client refnum out"=w245:refnum<k21>)  [unwired: 5 in]
                          }
                          frame 9 {
                            n138 = Index Array(array=w249) -> (element=w250:dbl)  [unwired: 1 in]
                            n139 = call-poly <vilib>:"Write.vi"("error in (no error)"=w251, "value"=w250, "node path"=w248, "OPC UA client refnum in"=w254) -> ("error out"=w252:errorcluster, "status"=w247:u32, "OPC UA client refnum out"=w253:refnum<k21>)  [unwired: 5 in]
                          }
                          frame 10 {
                            n140 = Index Array(array=w257) -> (element=w258:dbl)  [unwired: 1 in]
                            n141 = call-poly <vilib>:"Write.vi"("error in (no error)"=w259, "value"=w258, "node path"=w256, "OPC UA client refnum in"=w262) -> ("error out"=w260:errorcluster, "status"=w255:u32, "OPC UA client refnum out"=w261:refnum<k21>)  [unwired: 5 in]
                          }
                          frame 11 {
                            n142 = Index Array(array=w265) -> (element=w266:dbl)  [unwired: 1 in]
                            n143 = call-poly <vilib>:"Write.vi"("error in (no error)"=w267, "value"=w266, "node path"=w264, "OPC UA client refnum in"=w270) -> ("error out"=w268:errorcluster, "status"=w263:u32, "OPC UA client refnum out"=w269:refnum<k21>)  [unwired: 5 in]
                          }
                          frame 13 {
                            n144 = Index Array(array=w274) -> (element=w275:dbl)  [unwired: 1 in]
                            n145 = To Time Stamp(1:w275) -> (0:w273:timestamp)
                            n146 = call-poly <vilib>:"Write.vi"("error in (no error)"=w276, "value"=w273, "node path"=w272, "OPC UA client refnum in"=w279) -> ("error out"=w277:errorcluster, "status"=w271:u32, "OPC UA client refnum out"=w278:refnum<k21>)  [unwired: 5 in]
                          }
                          frame 101 {
                            n147 = To Unsigned Byte Integer(number=w283) -> (unsigned 8bit integer=w284:u8[])
                            n148 = Greater Than 0?(x=w284) -> (x > 0?=w282:bool[])
                            n149 = call-poly <vilib>:"Write.vi"("error in (no error)"=w285, "value"=w282, "node path"=w281, "OPC UA client refnum in"=w288) -> ("error out"=w286:errorcluster, "status"=w280:u32, "OPC UA client refnum out"=w287:refnum<k21>)  [unwired: 5 in]
                          }
                          frame 102 {
                            n150 = call-poly <vilib>:"Write.vi"("error in (no error)"=w292, "value"=w291, "node path"=w290, "OPC UA client refnum in"=w295) -> ("error out"=w293:errorcluster, "status"=w289:u32, "OPC UA client refnum out"=w294:refnum<k21>)  [unwired: 5 in]
                          }
                          frame 15, 103 {
                            n151 = call-poly <vilib>:"Write.vi"("error in (no error)"=w299, "value"=w298, "node path"=w297, "OPC UA client refnum in"=w302) -> ("error out"=w300:errorcluster, "status"=w296:u32, "OPC UA client refnum out"=w301:refnum<k21>)  [unwired: 5 in]
                          }
                          frame 104 {
                            n152 = call-poly <vilib>:"Write.vi"("error in (no error)"=w306, "value"=w305, "node path"=w304, "OPC UA client refnum in"=w309) -> ("error out"=w307:errorcluster, "status"=w303:u32, "OPC UA client refnum out"=w308:refnum<k21>)  [unwired: 5 in]
                          }
                          frame 105 {
                            n153 = call-poly <vilib>:"Write.vi"("error in (no error)"=w313, "value"=w312, "node path"=w311, "OPC UA client refnum in"=w316) -> ("error out"=w314:errorcluster, "status"=w310:u32, "OPC UA client refnum out"=w315:refnum<k21>)  [unwired: 5 in]
                          }
                          frame 106 {
                            n154 = call-poly <vilib>:"Write.vi"("error in (no error)"=w320, "value"=w319, "node path"=w318, "OPC UA client refnum in"=w323) -> ("error out"=w321:errorcluster, "status"=w317:u32, "OPC UA client refnum out"=w322:refnum<k21>)  [unwired: 5 in]
                          }
                          frame 107 {
                            n155 = call-poly <vilib>:"Write.vi"("error in (no error)"=w327, "value"=w326, "node path"=w325, "OPC UA client refnum in"=w330) -> ("error out"=w328:errorcluster, "status"=w324:u32, "OPC UA client refnum out"=w329:refnum<k21>)  [unwired: 5 in]
                          }
                          frame 108 {
                            n156 = call-poly <vilib>:"Write.vi"("error in (no error)"=w334, "value"=w333, "node path"=w332, "OPC UA client refnum in"=w337) -> ("error out"=w335:errorcluster, "status"=w331:u32, "OPC UA client refnum out"=w336:refnum<k21>)  [unwired: 5 in]
                          }
                          frame 109 {
                            n157 = call-poly <vilib>:"Write.vi"("error in (no error)"=w341, "value"=w340, "node path"=w339, "OPC UA client refnum in"=w344) -> ("error out"=w342:errorcluster, "status"=w338:u32, "OPC UA client refnum out"=w343:refnum<k21>)  [unwired: 5 in]
                          }
                          frame 110 {
                            n158 = call-poly <vilib>:"Write.vi"("error in (no error)"=w348, "value"=w347, "node path"=w346, "OPC UA client refnum in"=w351) -> ("error out"=w349:errorcluster, "status"=w345:u32, "OPC UA client refnum out"=w350:refnum<k21>)  [unwired: 5 in]
                          }
                          frame 111 {
                            n159 = call-poly <vilib>:"Write.vi"("error in (no error)"=w355, "value"=w354, "node path"=w353, "OPC UA client refnum in"=w358) -> ("error out"=w356:errorcluster, "status"=w352:u32, "OPC UA client refnum out"=w357:refnum<k21>)  [unwired: 5 in]
                          }
                          frame 113 {
                            n160 = To Time Stamp(1:w362) -> (0:w360:timestamp[])
                            n161 = call-poly <vilib>:"Write.vi"("error in (no error)"=w363, "value"=w360, "node path"=w361, "OPC UA client refnum in"=w366) -> ("error out"=w364:errorcluster, "status"=w359:u32, "OPC UA client refnum out"=w365:refnum<k21>)  [unwired: 5 in]
                          }
                        }
                        n162 = Set Variant Attribute(Variant=w172, name=w169, value=w171) -> (Variant out=w170:variant)  [unwired: 1 in, 2 out]
                      }
                    }
                  }
                }
                frame True {
                }
              }
              "Write Table" <- w124
              n163 = call <vilib>:"Async.Processes.Report.vi"("Error"=w107, "Process in"=w109) -> ("Stop"=w108:bool)  [unwired: 8 in, 1 out]
              n164 = Unbundle By Name(w107) -> ("code"=w111:i32)
              "Write Code" <- w111
              n165 = flat-sequence {
                tunnel: w107 -> [w135]
                tunnel: w122 -> [w134]
                tunnel: [w132] -> w121
                tunnel: [w131] -> w110
                tunnel: w108 -> [w130]
                frame #0 {
                  n166 = call "Global Stop Actions.vi"("error in (no error)"=w135, "Stop on Error?"=TRUE, "Stop?"=w130, "Stop Ref"=w134) -> ("error out"=w132:errorcluster, "Latched Stop"=w131:bool)  [unwired: 5 in, 1 out]
                }
              }
              n167 = Wait Until Next ms Multiple(millisecond multiple=u32 1) -> ()  [unwired: 1 out]
            }
            n168 = Compound Arithmetic op=OR(w49, w50, w51) -> (w48:bool)
            n169 = Merge Errors(w67, w78, w68) -> (w83:errorcluster)
            n170 = call "Poll.FormatErrorStatus.vi"("Read Table"=w55, "Write Table"=w52, "Read Code"=w54, "Write Code"=w53, "TotalTags"=w45) -> ("ErrorStatus"=w56:u32[])  [unwired: 5 in, 1 out]
            n171 = call-poly <vilib>:"Data.Processes.Execute.vi"("Values"=w56, "Ref"=w46) -> ()  [unwired: 9 in, 1 out]
          }
        }
      }
      frame Error {
        n172 = Unbundle By Name(w622) -> ("Process"=w621:refnum<class "Process.lvclass">)
        n173 = Unbundle By Name(w620) -> ("status"=w632:bool, "code"=w631:i32, "source"=w630:string)
        n174 = call <vilib>:"Async.Processes.Report.vi"("Error"=w620, "Stop Async on Error?"=FALSE ("Stop on Error?"), "Process in"=w621) -> ("Stop"=w619:bool)  [unwired: 7 in, 1 out]
        n175 = Format Into String(format string="%s,%d,%s,", w632, w631, w630) -> (resulting string=w628:string)  [unwired: 2 in, 1 out]
        n176 = Concatenate Strings("OPC Addon - Error" ("Message"), w628, "\r\n") -> (w626:string)
        n177 = call <vilib>:"NI VeriStand - Print Debug String.vi"("Message"=w626) -> ()  [unwired: 10 in, 1 out]
      }
    }
    n178 = Unbundle By Name(w25) -> ("Settings.PollEngine.Settings"=w24:T4[])
    n179 = Unbundle By Name(w23) -> ("Data Change"=w16:refnum<user-event>, "OPCEvent"=w17:refnum<event-registration>, "Stop Ref"=w19:refnum<data-value>, "SubscriptionIDs"=w22:u32[], "OPC UA client Ref"=w18:refnum<k21>)
    n180 = Wait Until Next ms Multiple(millisecond multiple=u32 100) -> ()  [unwired: 1 out]
    n181 = for {
      tunnel: w22 -> [w638] mode=indexing
      shift-right: [w639] -> w29
      shift-left: w18 -> [w640]
      tunnel: w24 -> [w637] mode=indexing
      tunnel: w30 -> [_]
      tunnel: [w635] -> w21 mode=indexing if=w633
      n182 = Unbundle By Name(w637) -> ("Tags"=w636:string[])
      n183 = Empty Array?(array=w636) -> (empty?=w634:bool)
      n184 = Not(x=w634) -> (.not. x?=w633:bool)
      n185 = case shown="False" w634 {
        tunnel: w640 -> [w645 w646]
        tunnel: [w644 w646] -> w639
        tunnel: w638 -> [w643 _]
        tunnel: w636 -> [w642 _]
        tunnel: [w641 _] -> w635
        frame False {
          n186 = call <vilib>:"Delete Monitored Nodes.vi"("array of node path"=w642, "subscription ID in"=w643, "OPC UA client refnum in"=w645) -> ("subscription ID out"=w641:u32, "OPC UA client refnum out"=w644:refnum<k21>)  [unwired: 5 in, 2 out]
        }
        frame True {
        }
      }
    }
    n187 = call <vilib>:"Delete Subscriptions.vi"("array of subscription ID"=w21, "OPC UA client refnum in"=w29) -> ("OPC UA client refnum out"=w31:refnum<k21>)  [unwired: 7 in, 2 out]
    n188 = call <vilib>:"Disconnect.vi"("OPC UA client refnum in"=w31) -> ("error out"=→"error out":errorcluster)  [unwired: 10 in]
    n189 = Unregister For Events(event registration refnum=w17) -> ()  [unwired: 1 in, 1 out]
    n190 = Delete Data Value Reference(data value reference=w19) -> ()  [unwired: 1 in, 2 out]
    n191 = Destroy User Event(user event=w16) -> ()  [unwired: 1 in, 1 out]
  }
